vi "Write Hardware.vi"(8 "error in (no error)":errorcluster, 10 "command":string, 11 "Instrument in":refnum<class "Instrument.lvclass">) -> (0 "error out":errorcluster, 3 "Instrument out":refnum<class "Instrument.lvclass">)   [LabVIEW 2019, in "Instrument.lvlib" / "Instrument.lvclass"]
doc: "Override <b>Write Hardware</b> to write to your instrument hardware."
uses:
  Instrument.lvclass
  Instrument.lvclass/Instrument.ctl
  subsystems/HAL/HAL.lvclass
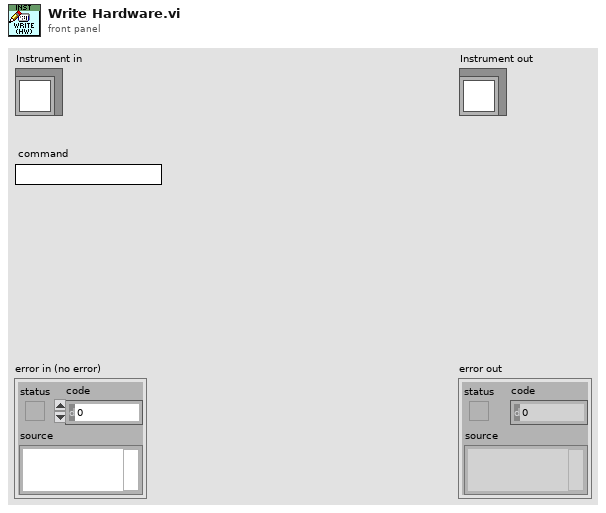
[diagram p1: front panel]
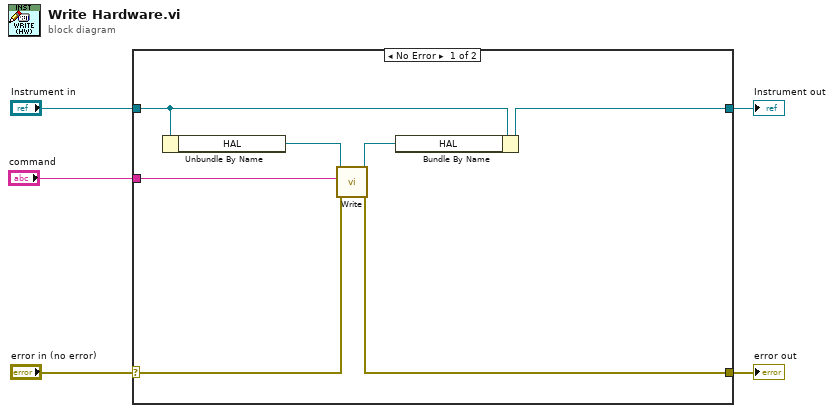
[diagram p0: block diagram]
diagram:
  n1 = case shown="No Error" "error in (no error)" {
    selector: "error in (no error)" -> [w10 w14]
    tunnel: [w9 w14] -> w4
    tunnel: [w7 w13] -> w2
    tunnel: "Instrument in" -> [w6 w13]
    tunnel: "command" -> [w11 _]
    frame No Error {
      n2 = Unbundle By Name(w6) -> ("HAL"=w12:refnum<class "HAL.lvclass">)
      n3 = call-dynamic "Write.vi"("error in (no error)"=w10, "command"=w11, "HAL in"=w12) -> ("error out"=w9:errorcluster, "HAL out"=w8:refnum<class "HAL.lvclass">)  [unwired: 7 in]
      n4 = Bundle By Name(cluster=w6, "HAL"=w8) -> (w7:refnum<class "Instrument.lvclass">)
    }
    frame Error {
    }
  }
  "error out" <- w4
  "Instrument out" <- w2
